vi "ReadRaw.vi"() -> ()   [LabVIEW 2015]
uses:
  <vilib>/FPGAPlugInAG/USB-7855R OEM/niLvFpga_Open_USB-7855R OEM.vi
  <vilib>/rvi/interface/common/dynamic/niFpgaDynamicAddResources.vi
  <vilib>/Utility/error.llb/Error Cluster From Error Code.vi
  <vilib>/rvi/errors/niLvFpgaAdjustHostInterfaceError.vi
  <vilib>/measure/matone.llb/Extract Single Tone Information 1 Chan.vi
  <vilib>/FPGAPlugInAG/Dynamic/niLvFpga_Close_Dynamic.vi
  <vilib>/rvi/interface/nirviOpenFPGA/nirviOpenFPGA.xnode
  FPGA Bitfiles/DloopFunds_FPGATarget_Read_4KnPo7fuNVg.lvbitx
  SendRaw.vi
  <vilib>/rvi/interface/nirviReadWriteControl/nirviReadWriteControl.xnode
  <vilib>/rvi/interface/nirviMethod/nirviMethod.xnode
  <vilib>/rvi/interface/nirviCloseFPGA/nirviCloseFPGA.xnode
  <vilib>/Analysis/NI_AALPro.lvlib
  <vilib>/measure/NI_MAPro.lvlib
  <vilib>/FPGAPlugInAG/Dynamic/niLvFpga_ReadFifo_Dynamic.vi
  <vilib>/rvi/errors/niLvFpgaMergeErrorWithErrorCode.vi
  NiFpgaLv.dll
  <vilib>/rvi/interface/Simulation/niFpgaSimulationCallBeginRW.vi
panel:
  out "Frequ":dbl
  in  "Channel":i16
  in  "Raw":bool
  out "Output time":dbl
  in  "Peak height":fxp<+/-,16,4>
  in  "Stop at peak":bool
  in  "Input Period (ticks)":i16=80
  out "Signal":dynamicdata(graph)
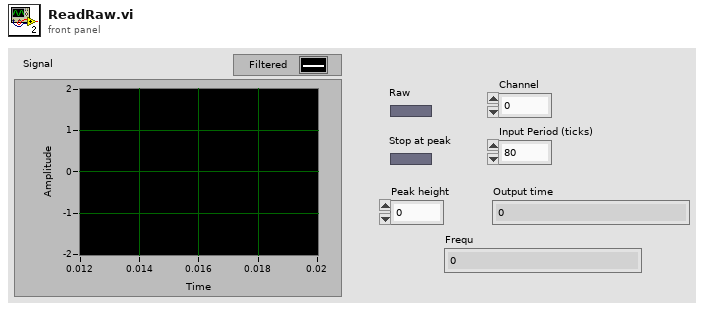
[diagram p1: front panel]
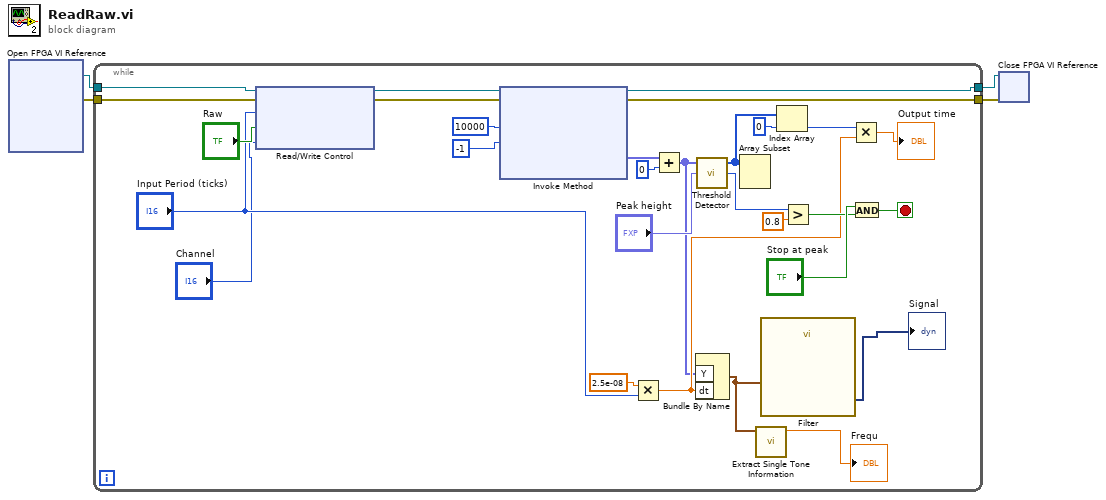
[diagram p0: block diagram]
diagram:
  n1 = xnode "Open FPGA VI Reference"() -> ("FPGA VI Reference Out"=w2:refnum<k20>, "error out"=w1:errorcluster)  [unwired: 2 in]
  n2 = while {
    tunnel: [w26] -> w4
    tunnel: [w32] -> w3
    tunnel: w2 -> [w30]
    tunnel: w1 -> [w29]
    stop <- w24 stop-if-true
    n3 = xnode "Read/Write Control"("FPGA VI Reference In"=w30, "error in"=w29, "Input period (ticks)"="Input Period (ticks)", "Raw"="Raw", "Channel"="Channel") -> ("FPGA VI Reference Out"=w27:refnum<k20>, "error out"=w28:errorcluster)
    n4 = xnode "Invoke Method"("FPGA VI Reference In"=w27, "error in"=w28, "Number of Elements"=10000, "Timeout (ms)"=-1) -> ("FPGA VI Reference Out"=w26:refnum<k20>, "error out"=w32:errorcluster, "Data"=w14:fxp<+/-,24,16>[])  [unwired: 1 out]
    n5 = Multiply(x=2.5e-08, y="Input Period (ticks)") -> (x*y=w16:dbl)
    n6 = Add(x=w14, y=0) -> (x+y=w13:fxp<+/-,41,33>[])
    n7 = Bundle By Name("Y"=w13, "dt"=w16) -> (w7:waveform(dbl))  [unwired: 1 in]
    n8 = call <vilib>:"Threshold Detector.vi"("threshold"="Peak height", "X"=w13) -> ("count"=w21:i32, "Indices"=w9:i32[])  [unwired: 1 in, 1 out]
    n9 = Array Subset(array=w9) -> ()  [unwired: 2 in, 1 out]
    n10 = call-poly <vilib>:"Extract Single Tone Information.vi"("time signal in"=w7) -> ("detected frequency"=→"Frequ":dbl)  [unwired: 5 in, 5 out]
    n11 = call "Filter"("Signal"=w7) -> ("Filtered Signal"=→"Signal":dynamicdata)  [unwired: 9 in, 1 out]
    n12 = Index Array(array=w9, index=0) -> (element=w17:i32)
    n13 = Greater?(x=w21, y=0.8) -> (0:w19:bool)
    n14 = Multiply(x=w17, y=w16) -> (x*y=→"Output time":dbl)
    n15 = And(x="Stop at peak", y=w19) -> (x .and. y?=w24:bool)
  }
  n16 = xnode "Close FPGA VI Reference"("FPGA VI Reference In"=w4, "error in"=w3) -> ()  [unwired: 1 out]
